vi "class_data.vi"() -> ()   [LabVIEW 2010]
uses:
  System.Windows.Forms
panel:
  out "Event Registration reference":refnum<event-registration>
  out "NotifyIcon reference":refnum<k24>
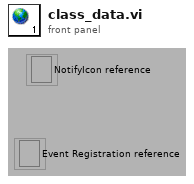
[diagram p1: front panel]
diagram:
